vi "SimpleBuilder.vi"() -> ()   [LabVIEW 2019]
uses:
  labview source/gRPC lv Support/Server API/typeDefs/Message Element Type.ctl
  labview source/gRPC lv Support/Server API/typeDefs/Message Metadata.ctl
  labview source/gRPC lv Support/Server API/typeDefs/Message Element Metadata.ctl
  50cd6ca9-b915-40c5-a5da-5a0bdd109e0e.vi
  b10376ed-0ca3-44e2-870d-a1c3b67942c2.vi
  labview source/gRPC lv Support/Server API/Translate Protobuf Error.vi
  <vilib>/AdvancedString/1D String Array to Delimited String.vi
  labview source/gRPC lv Support/Server API/Server/Get Server DLL Path.vi
  labview source/gRPC lv Support/grpc-lvsupport.lvlib
panel:
  out "Numeric":i32
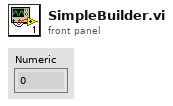
[diagram p1: front panel]
types:
  T1 = typedef "grpc-lvsupport.lvlib/Message Metadata.ctl" = cluster{"Version":i32, "Name":string, "Type Url":string, "Elements":T2[]}
  T2 = typedef "grpc-lvsupport.lvlib/Message Element Metadata.ctl" = cluster{"Embedded Message Name":string, "Protobuf Index":i32, "MessageElementType":T3, "Repeated":bool}
  T3 = typedef "grpc-lvsupport.lvlib/Message Element Type.ctl" = enum32{"Int32Value", "FloatValue", "DoubleValue", "BoolValue", "StringValue", "MessageValue", "Int64Value", "UInt32Value", "UInt64Value", "EnumValue", "Bytes", "Fixed64", "Fixed32", "SFixed64", "SFixed32", "SInt64", "SInt32"}
  T4 = typedef "grpc-lvsupport.lvlib/grpcId.ctl" = u64
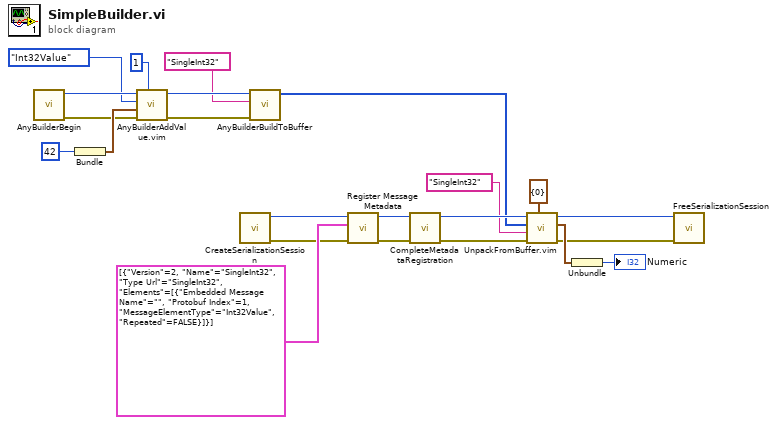
[diagram p0: block diagram]
diagram:
  n1 = call "AnyBuilderBegin.vi"() -> ("error out"=w6:errorcluster, "Builder Ref Out"=w23:T4)  [unwired: 9 in]
  n2 = Bundle(42) -> (w20:cluster{i32})  [unwired: 1 in]
  n3 = call "AnyBuilderAddValue.vim"("protobufId"=1, "error in"=w6, "Value"=w20, "MessageElementType"=Message_Element_Type."Int32Value", "gRPCid in"=w23) -> ("error out"=w5:errorcluster, "gRPCid out"=w14:u64)  [unwired: 5 in]
  n4 = call "CreateSerializationSession.vi"() -> ("error out"=w4:errorcluster, "Serialization Session ID"=w18:T4)  [unwired: 10 in]
  n5 = call "AnyBuilderBuildToBuffer.vi"("error in"=w5, "Message Type"="SingleInt32", "Builder Ref"=w14) -> ("Buffer"=w8:u8[])  [unwired: 7 in, 1 out]
  n6 = call "Register Message Metadata.vi"("error in"=w4, "Messages"=T1[] [{"Version"=2, "Name"="SingleInt32", "Type Url"="SingleInt32", "Elements"=[{"Embedded Message Name"="", "Protobuf Index"=1, "MessageElementType"=enum."Int32Value", "Repeated"=FALSE}]}], "gRPCid in"=w18) -> ("error out"=w3:errorcluster, "gRPCid out"=w16:T4)  [unwired: 7 in]
  n7 = call "CompleteMetadataRegistration.vi"("error in"=w3, "gRPC ID in"=w16) -> ("error out"=w2:errorcluster, "gRPC ID Out"=w10:T4)  [unwired: 8 in]
  n8 = call "UnpackFromBuffer.vim"("Data Type"=cluster{i32} {0}, "error in"=w2, "Message Type"="SingleInt32", "Buffer"=w8, "gRPCid in"=w10) -> ("error out"=w1:errorcluster, "Unpacked Value"=w11:cluster{i32}, "gRPCid out"=w7:u64)  [unwired: 4 in]
  n9 = Unbundle(w11) -> (→"Numeric":i32)
  n10 = call "FreeSerializationSession.vi"("error in"=w1, "Serialization Session ID"=w7) -> ()  [unwired: 9 in, 1 out]
